vi "Part 1.vi"(11 "Input":string) -> (3 "Output":i64)   [LabVIEW 2021]
uses:
  <userlib>/_OpenG.lib/string/string.llb/Convert EOLs (String)__ogtk.vi
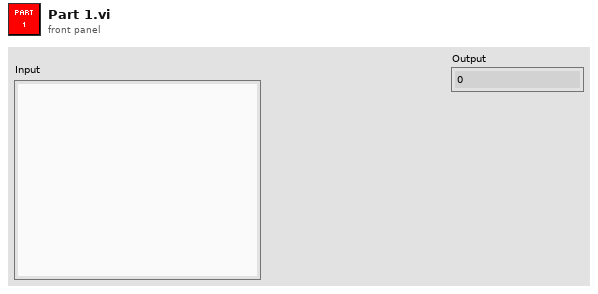
[diagram p1: front panel]
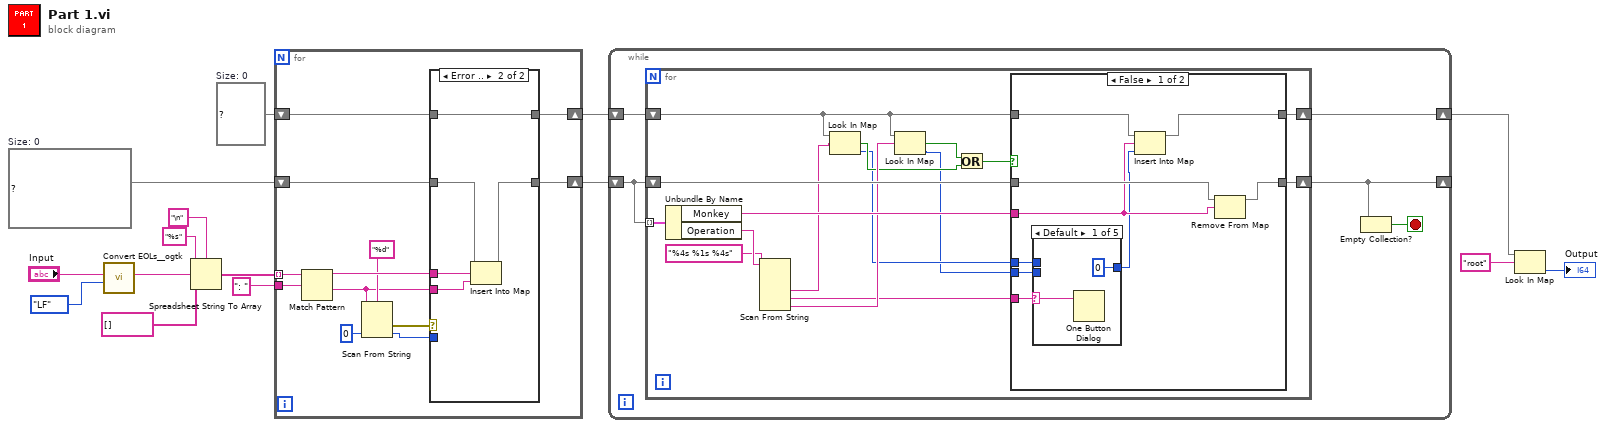
[diagram p0: block diagram]
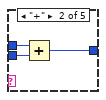
[diagram p2: hidden frame]
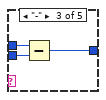
[diagram p3: hidden frame]
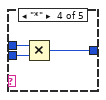
[diagram p4: hidden frame]
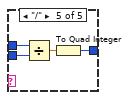
[diagram p5: hidden frame]
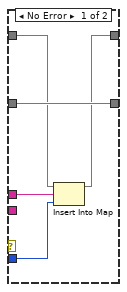
[diagram p7: hidden frame]
diagram:
  w6 = map{string, i64} {}  # Size: 0
  w7 = map{string, string} {}  # Size: 0
  n1 = call-poly <userlib>:"Convert EOLs__ogtk.vi"("Convert to:"=enum16{"CR", "LF", "CRLF"}."LF", "String in"="Input") -> ("String out"=w11:string)  [unwired: 9 in]
  n2 = Spreadsheet String To Array(delimiter (Tab)="\n", format string="%s", spreadsheet string=w11, array type (2D Dbl)=string[] []) -> (array=w9:string[])
  n3 = for {
    tunnel: w9 -> [w27] mode=indexing
    shift-right: [w23] -> w1
    shift-left: w7 -> [w24]
    tunnel: ": " -> [w26]
    shift-right: [w18] -> w3
    shift-left: w6 -> [w19]
    n4 = Match Pattern(string=w27, regular expression=w26) -> (before substring=w25:string, after substring=w16:string)  [unwired: 1 in, 2 out]
    n5 = Scan From String(format string="%d", input string=w16, default 1=i64 0 ("default value 1")) -> (error out=w20:errorcluster, output 1=w17:i64)  [unwired: 2 in, 2 out]
    n6 = case shown="Error .." w20 {
      tunnel: w25 -> [w31 w37]
      tunnel: w24 -> [w32 w36]
      tunnel: [w32 w35] -> w23
      tunnel: w19 -> [w30 w34]
      tunnel: [w29 w34] -> w18
      tunnel: w17 -> [w28 _]
      tunnel: w16 -> [_ w33]
      frame No Error {
        n7 = Insert Into Map(map in=w30, key=w31, value=w28) -> (map out=w29:map{string, i64})  [unwired: 2 out]
      }
      frame Error {
        n8 = Insert Into Map(map in=w36, key=w37, value=w33) -> (map out=w35:map{string, string})  [unwired: 2 out]
      }
    }
  }
  n9 = while {
    shift-right: [w40] -> w2
    shift-left: w3 -> [w41]
    shift-right: [w38] -> _
    shift-left: w1 -> [w39]
    stop <- w42 stop-if-true
    n10 = for {
      tunnel: w39 -> [w55] mode=indexing
      shift-right: [w56] -> w40
      shift-left: w41 -> [w50]
      shift-right: [w57] -> w38
      shift-left: w39 -> [w58]
      n11 = Unbundle By Name(w55) -> ("Monkey"=w54:string, "Operation"=w53:string)
      n12 = Scan From String(format string="%4s %1s %4s", input string=w53) -> (output 1=w51:string, output 2=w45:string, output 3=w49:string)  [unwired: 5 in, 3 out]
      n13 = Look In Map(map=w50, key=w51) -> (key not found?=w47:bool, value=w44:i64)  [unwired: 1 in]
      n14 = Look In Map(map=w50, key=w49) -> (key not found?=w48:bool, value=w43:i64)  [unwired: 1 in]
      n15 = Or(x=w48, y=w47) -> (x .or. y?=w46:bool)
      n16 = case shown="False" w46 {
        tunnel: w58 -> [w66 w83]
        tunnel: [w67 w83] -> w57
        tunnel: w50 -> [w64 w84]
        tunnel: [w65 w84] -> w56
        tunnel: w54 -> [w63 _]
        tunnel: w45 -> [w62 _]
        tunnel: w44 -> [w61 _]
        tunnel: w43 -> [w60 _]
        frame False {
          n17 = case shown="Default" w62 {
            selector: w62 -> [w68 _ _ _ _]
            tunnel: w61 -> [_ w72 w75 w78 w82]
            tunnel: w60 -> [_ w71 w74 w77 w81]
            tunnel: [i64 0 w70 w73 w76 w79] -> w59
            frame Default {
              n18 = One Button Dialog(message=w68) -> ()  [unwired: 1 in, 1 out]
            }
            frame "+" {
              n19 = Add(x=w72, y=w71) -> (x+y=w70:i64)
            }
            frame "-" {
              n20 = Subtract(x=w75, y=w74) -> (x-y=w73:i64)
            }
            frame "*" {
              n21 = Multiply(x=w78, y=w77) -> (x*y=w76:i64)
            }
            frame "/" {
              n22 = Divide(x=w82, y=w81) -> (x/y=w80:dbl)
              n23 = To Quad Integer(1:w80) -> (0:w79:i64)
            }
          }
          n24 = Insert Into Map(map in=w64, key=w63, value=w59) -> (map out=w65:map{string, i64})  [unwired: 2 out]
          n25 = Remove From Map(10:w63, 11:w66) -> (3:w67:map{string, string})  [unwired: 2 out]
        }
        frame True {
        }
      }
    }
    n26 = Empty Collection?(1:w38) -> (0:w42:bool)
  }
  n27 = Look In Map(map=w2, key="root") -> (value=→"Output":i64)  [unwired: 1 in, 1 out]
